vi "test Basic Formatting.vi"(8 "error in (no error)":errorcluster, 11 "TestCase in":refnum<class "UUID Structure Tests.lvclass">) -> (0 "error out":errorcluster, 3 "TestCase out":refnum<class "UUID Structure Tests.lvclass">)   [LabVIEW 2015, in "UUID Structure Tests.lvclass"]
uses:
  UUID Structure Tests.lvclass
  <vilib>/addons/_JKI Toolkits/VI Tester/TestCase.llb/TestCase.lvclass
  UUID/UUID.lvclass
  <vilib>/Wiresmith Technology/VITAC (VI Tester Advanced Comparisons)/VITAC.lvlib
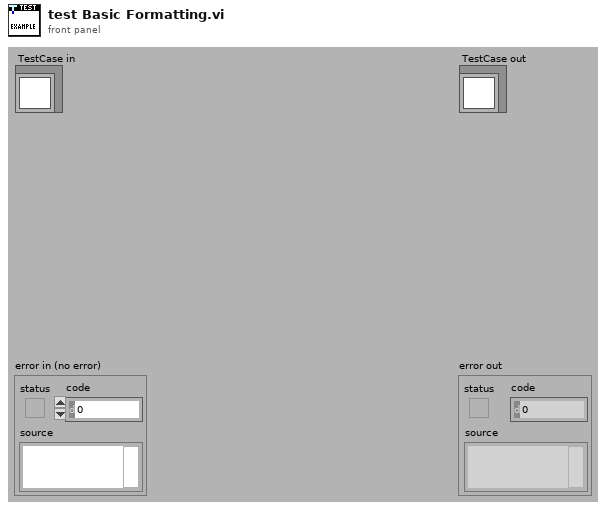
[diagram p1: front panel]
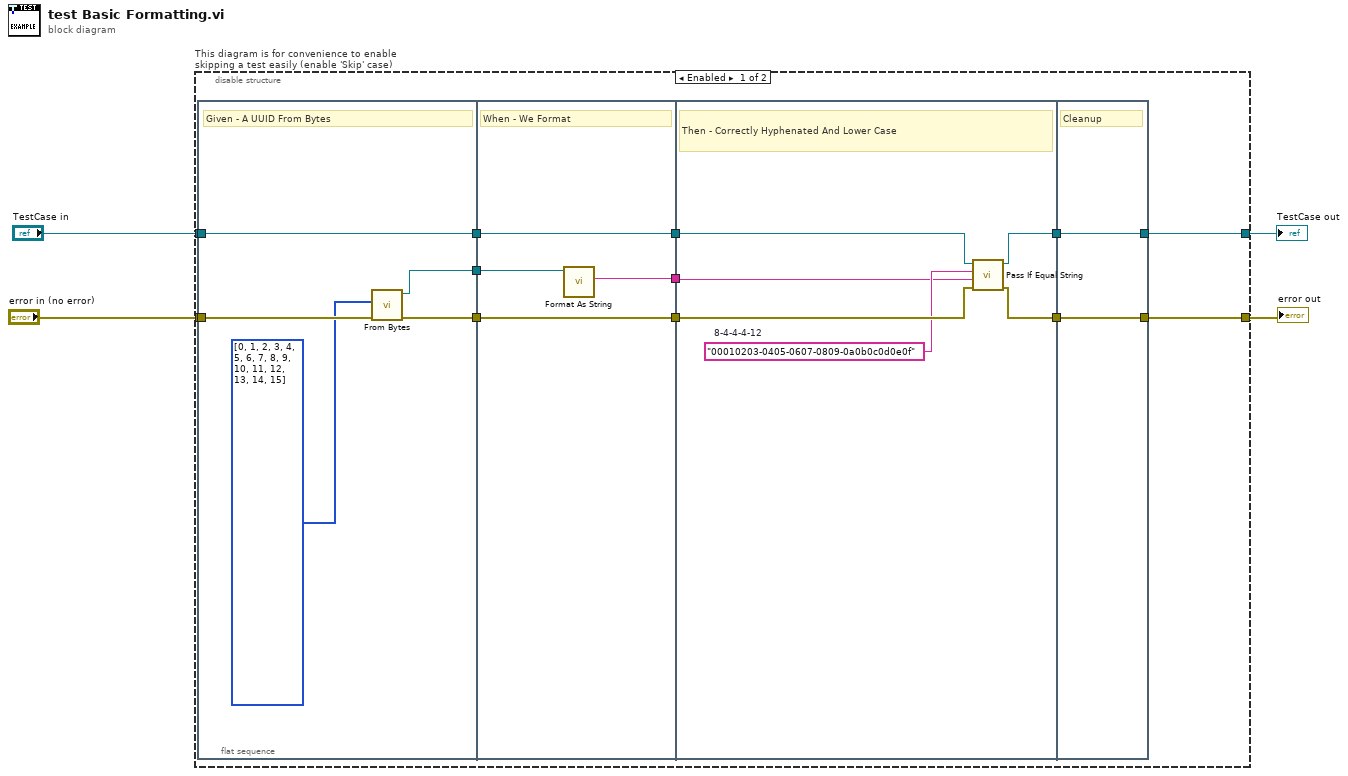
[diagram p0: block diagram]
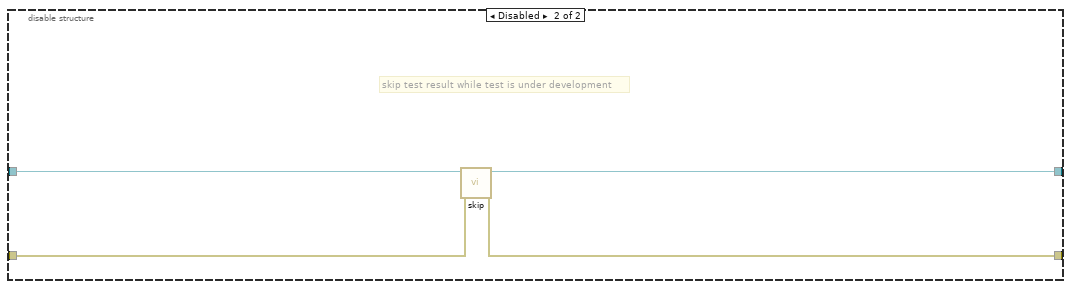
[diagram p2: hidden frame]
diagram:
  n1 = disable-structure "This diagram is for convenience to enable skipping a test easily (enable 'Skip' case)" shown="Enabled" {
    disable-tunnel: "TestCase in" -> [w10 w37]
    disable-tunnel: [w8 w35] -> w1
    disable-tunnel: [w7 w36] -> w3
    disable-tunnel: "error in (no error)" -> [w9 w34]
    frame Enabled {
      n2 = flat-sequence {
        tunnel: w9 -> [w20]
        tunnel: w10 -> [w21]
        tunnel: [w21] -> w16
        tunnel: [w19] -> w15
        tunnel: [w18] -> w6
        tunnel: [w25] -> w14
        tunnel: [w24] -> w13
        tunnel: w16 -> [w25]
        tunnel: w15 -> [w24]
        tunnel: w6 -> [w23]
        tunnel: [w22] -> w5
        tunnel: [w30] -> w12
        tunnel: [w28] -> w11
        tunnel: w14 -> [w31]
        tunnel: w13 -> [w29]
        tunnel: w5 -> [w26]
        tunnel: [w32] -> w7
        tunnel: [w33] -> w8
        tunnel: w12 -> [w33]
        tunnel: w11 -> [w32]
        frame #0 {
          # "Given - A UUID From Bytes"
          n3 = call "From Bytes.vi"("error in (no error)"=w20, "Bytes"=u8[] [0, 1, 2, 3, 4, 5, 6, 7, 8, 9, 10, 11, 12, 13, 14, 15]) -> ("error out"=w19:errorcluster, "UUID out"=w18:refnum<class "UUID.lvclass">)  [unwired: 8 in]
        }
        frame #1 {
          # "When - We Format"
          n4 = call "Format As String.vi"("UUID.lvclass"=w23) -> ("String"=w22:string)  [unwired: 10 in]
        }
        frame #2 {
          w27 = "00010203-0405-0607-0809-0a0b0c0d0e0f"  # 8-4-4-4-12
          # "Then - Correctly Hyphenated And Lower Case"
          n5 = call <vilib>:"Pass If Equal String.vi"("error in (no error)"=w29, "actual"=w26, "expected"=w27, "TestCase in"=w31) -> ("error out"=w28:errorcluster, "TestCase out"=w30:refnum<class "UUID Structure Tests.lvclass">)  [unwired: 6 in]
        }
        frame #3 {
          # "Cleanup"
        }
      }
    }
    frame Disabled {
      # "skip test result while test is under development"
      n6 = call <vilib>:"skip.vi"("error in (no error)"=w34, "TestCase in"=w37) -> ("error out"=w36:errorcluster, "TestCase out"=w35:refnum<class "UUID Structure Tests.lvclass">)  [unwired: 8 in]
    }
  }
  "error out" <- w3
  "TestCase out" <- w1
